vi "Set Working Directory.vi"(8 "error in (no error)":errorcluster caption="entrée d'erreur (pas d'erreur)", 10 "Working Directory":string, 11 "Class Instrument Process en entrée":refnum<class "Class Instrument Process.lvclass">) -> (0 "error out":errorcluster caption="sortie d'erreur", 3 "Class Instrument Process en sortie":refnum<class "Class Instrument Process.lvclass">)   [LabVIEW 2020, in "Library Instrument & Equipement.lvlib" / "Library Instruments.lvlib" / "Class Instrument Process.lvclass"]
uses:
  Class Instrument Process.lvclass
  Class Instrument Process.lvclass/Class Instrument Process.ctl
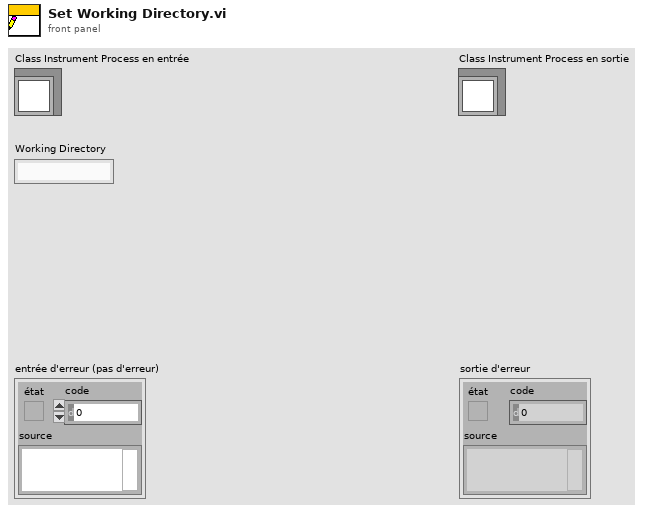
[diagram p1: front panel]
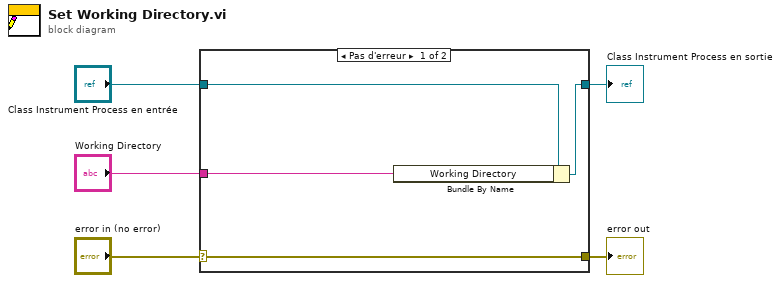
[diagram p0: block diagram]
diagram:
  n1 = case shown="Pas d'erreur" "error in (no error)" {
    selector: "error in (no error)" -> [w9 w10]
    tunnel: [w9 w10] -> w4
    tunnel: [w7 w11] -> w2
    tunnel: "Class Instrument Process en entrée" -> [w8 w11]
    tunnel: "Working Directory" -> [w6 _]
    frame No Error {
      n2 = Bundle By Name(cluster=w8, "Working Directory"=w6) -> (w7:refnum<class "Class Instrument Process.lvclass">)
    }
    frame Error {
    }
  }
  "error out" <- w4
  "Class Instrument Process en sortie" <- w2
